vi "Prompt Import 3rd Party ECAT Slaves Will Reboot.vi"() -> (3 "Continue?":bool)   [LabVIEW 2019, in "SEECD System Explorer.lvlib"]
uses:
  SEECD System Explorer.lvlib
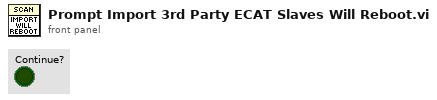
[diagram p1: front panel]
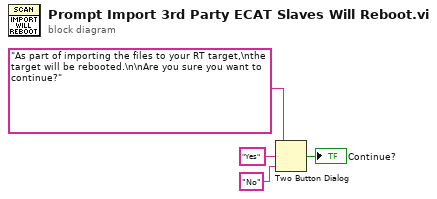
[diagram p0: block diagram]
diagram:
  n1 = Two Button Dialog(message="As part of importing the files to your RT target,\nthe target will be rebooted.\n\nAre you sure you want to continue?", 1:"No" ("F button name (\"Cancel\")"), 2:"Yes" ("T button name (\"OK\")")) -> (T button?=→"Continue?":bool)
